vi "objTracker.vi"() -> ()   [LabVIEW 2012]
uses:
  <userlib>/ImageProcessing/InitCamera_NTSC.vi
  <userlib>/ImageProcessing/FilterBluePlane.vi
  <userlib>/ImageProcessing/FilterRedPlane.vi
panel:
  in  "B Color 2":i16(slide)=200 scale=0.0..255.0
  in  "G Color 2":i16(slide)=36 scale=0.0..255.0
  in  "R Color 2":i16(slide)=100 scale=0.0..255.0
  out "image 3":picture
  in  "B Color":i16(slide)=200 scale=0.0..255.0
  in  "G Color":i16(slide)=36 scale=0.0..255.0
  in  "R Color":i16(slide)=100 scale=0.0..255.0
  out "image 2":picture
  in  "blue threshold":cluster{u8, u8}(slide)={0, 44} scale=0.0..255.0
  in  "red threshold":cluster{u8, u8}(slide)={115, 255} scale=0.0..255.0
  out "image":picture
  in  "Stop":bool
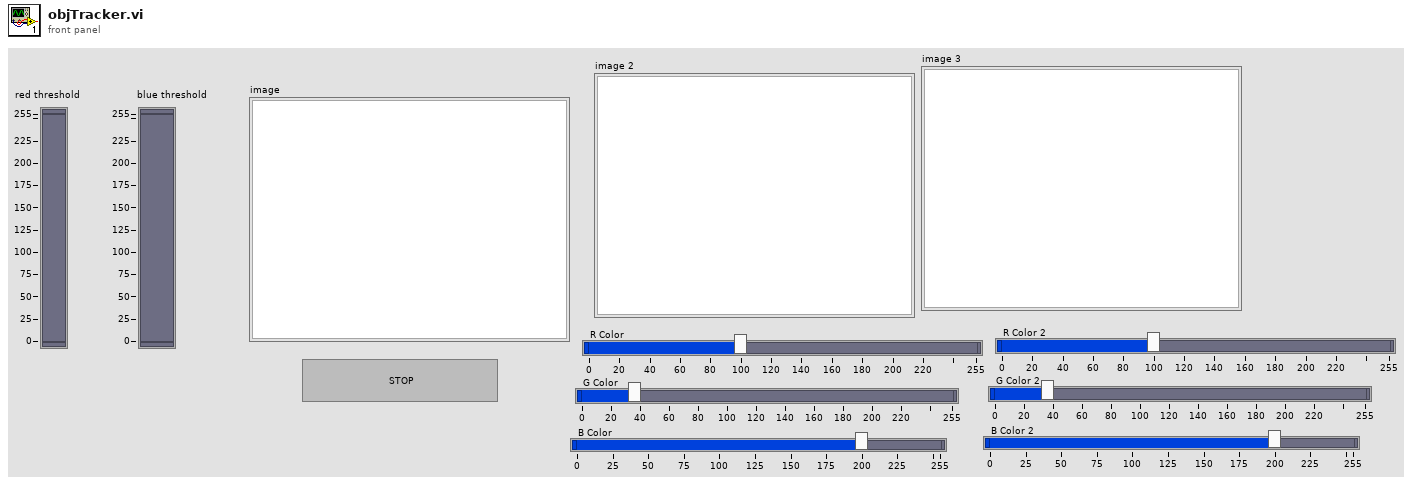
[diagram p1: front panel]
types:
  T1 = typedef "QT_Ref.ctl" = refnum<k1>
  T2 = typedef "QT_Image.ctl" = cluster{"Width":i32, "Height":i32, "Depth":i32, "data":u8[], "Compressed data":u8[], "Color table":u32[], "Duration":i32, "Options":i32, "Timestamp":i32, "ID":i32, "Reserved":i32, "Dialogs":u32}
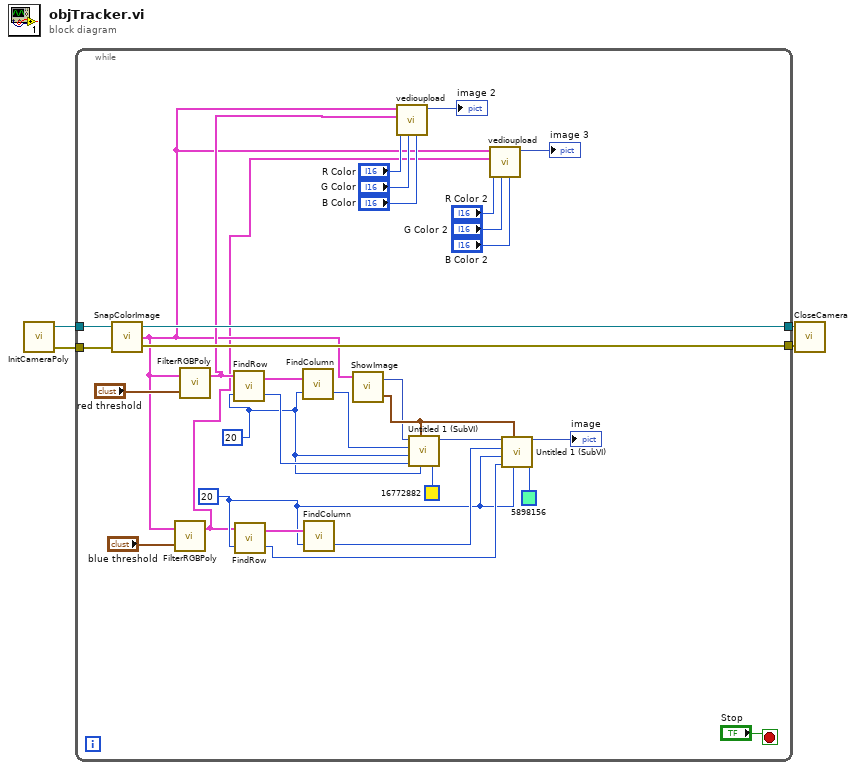
[diagram p0: block diagram]
diagram:
  n1 = call-poly <userlib>:"InitCameraPoly.vi"() -> ("error out"=w1:errorcluster, "QT Ref Out"=w2:T1)  [unwired: 2 in]
  n2 = while {
    tunnel: w1 -> [w36]
    tunnel: w2 -> [w35]
    tunnel: [w34] -> w3
    tunnel: [w33] -> w4
    stop <- "Stop" stop-if-true
    w16 = i8 20 ("# Columns")
    w19 = i8 20 ("# Rows")
    n3 = call <userlib>:"SnapColorImage.vi"("error in (no error)"=w36, "QT Ref In"=w35) -> ("error out"=w34:errorcluster, "Image Out"=w6:T2, "QT Ref Out"=w33:T1)  [unwired: 1 in]
    n4 = call-poly <userlib>:"FilterRGBPoly.vi"("threshold"="blue threshold", "Image in"=w6) -> ("Image out"=w5:T2)  [unwired: 1 out]
    n5 = call-poly <userlib>:"FilterRGBPoly.vi"("threshold"="red threshold", "Image in"=w6) -> ("Image out"=w11:T2)  [unwired: 1 out]
    n6 = call <userlib>:"FindRow.vi"("# Rows"=w19, "Image In"=w11) -> ("Row"=w20:i32, "Image Out"=w29:T2)
    n7 = call <userlib>:"FindRow.vi"("# Rows"=w16, "Image In"=w5) -> ("Row"=w17:i32, "Image Out"=w28:T2)
    n8 = call <userlib>:"FindColumn.vi"("# Columns"=w19, "Image In"=w29) -> ("Column"=w21:i32)  [unwired: 1 out]
    n9 = call <userlib>:"FindColumn.vi"("# Columns"=w16, "Image In"=w28) -> ("Column"=w18:i32)  [unwired: 1 out]
    n10 = call <userlib>:"ShowImage.vi"("Image"=w6) -> ("dimensions"=w25:cluster{"Width":i32, "Height":i32}, "image"=w22:picture)  [unwired: 2 in]
    n11 = call "vedioupload.vi"("B Color"="B Color", "G Color"="G Color", "R Color"="R Color", "Mask In"=w11, "Original Image"=w6) -> ("image Out"=→"image 2":picture)  [unwired: 6 in]
    n12 = call "Untitled 1 (SubVI).vi"("color(black)"=u32 16772882, "# Rows"=w19, "dimensions"=w25, "Row"=w20, "# Columns"=w19, "Column"=w21, "image"=w22) -> ("new picture"=w23:picture)  [unwired: 4 in]
    n13 = call "vedioupload.vi"("B Color"="B Color 2", "G Color"="G Color 2", "R Color"="R Color 2", "Mask In"=w5, "Original Image"=w6) -> ("image Out"=→"image 3":picture)  [unwired: 6 in]
    n14 = call "Untitled 1 (SubVI).vi"("color(black)"=u32 5898156, "# Rows"=w16, "dimensions"=w25, "Row"=w17, "# Columns"=w16, "Column"=w18, "image"=w23) -> ("new picture"=→"image":picture)  [unwired: 4 in]
  }
  n15 = call <userlib>:"CloseCamera.vi"("error in (no error)"=w3, "QT Ref In"=w4) -> ()  [unwired: 1 in, 1 out]
